vi "Stop Data Grid.vi"(8 "error in (no error)":errorcluster, 11 "DataGridView in":refnum<class "DataGridView.lvclass">) -> (0 "error out":errorcluster, 3 "DataGridView out":refnum<class "DataGridView.lvclass">)   [LabVIEW 2016, in "DataGrid.lvlib" / "DataGridView.lvclass"]
doc: "This VI must be called to properly stop the grid, as it unregisters the .net callback events, that otherwise, stay running and lock the classes."
uses:
  <userlib>/LabVIEWdotNetDataGrid/source/DataGridView/DataGridView.lvclass
  <userlib>/LabVIEWdotNetDataGrid/source/DataGridView/DataGridView.lvclass/DataGridView.ctl
  System.Windows.Forms
  <userlib>/LabVIEWdotNetDataGrid/source/DataTable/DataTable.lvclass/DataTable.ctl
  System.Data
  <userlib>/LabVIEWdotNetDataGrid/source/DataTable/Read DataTable.vi
  <userlib>/LabVIEWdotNetDataGrid/source/DataTable/DataTable.lvclass
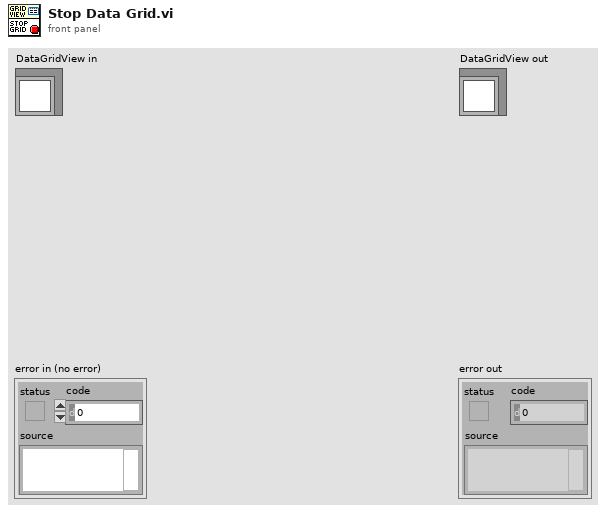
[diagram p1: front panel]
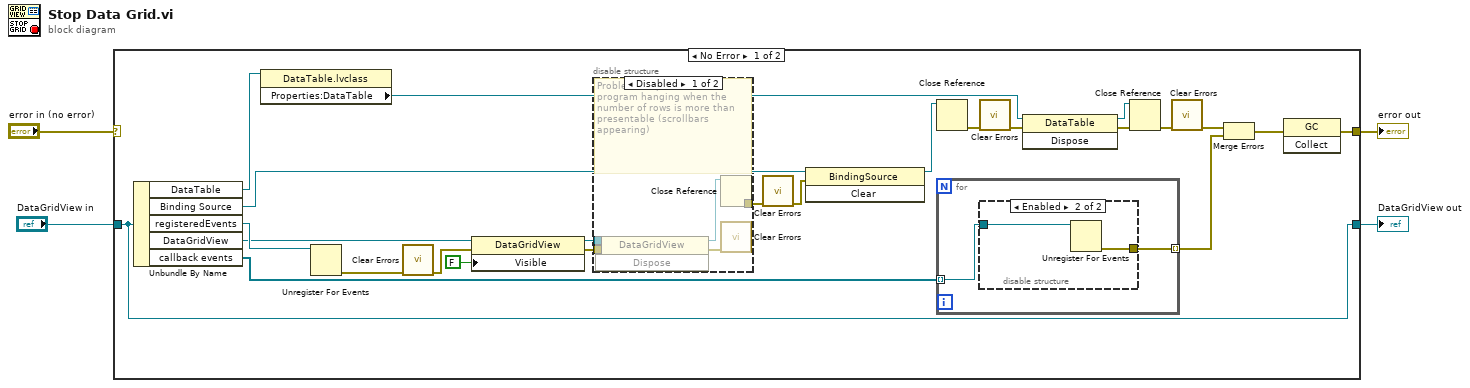
[diagram p0: block diagram]
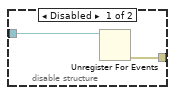
[diagram p3: hidden frame]
diagram:
  n1 = case shown="No Error" "error in (no error)" {
    selector: "error in (no error)" -> [_ w42]
    tunnel: [w24 w42] -> w3
    tunnel: [w28 w41] -> w1
    tunnel: "DataGridView in" -> [w28 w41]
    frame No Error {
      n2 = Unbundle By Name(w28) -> ("DataTable"=w23:refnum<class "DataTable.lvclass">, "Binding Source"=w20:refnum<k24>, "registeredEvents"=w22:refnum<event-registration>, "DataGridView"=w21:refnum<k24>, "callback events"=w27:refnum<k27>[])
      n3 = property class="DataTable.lvclass"(reference=w23) -> ("Properties:DataTable"=w19:refnum<k24>)  [unwired: 1 in, 2 out]
      n4 = Unregister For Events(event registration refnum=w22) -> (error out=w16:errorcluster)  [unwired: 1 in]
      n5 = call <vilib>:"Clear Errors.vi"("error in (no error)"=w16) -> ("error out"=w6:errorcluster)  [unwired: 5 in, 1 out]
      n6 = property class="DataGridView"(reference=w21, error in=w6, "Visible"=FALSE) -> (reference out=w14:refnum<k24>, error out=w13:errorcluster)
      n7 = disable-structure shown="Disabled" {
        disable-tunnel: w14 -> [w32 _]
        disable-tunnel: w13 -> [w31 w34]
        disable-tunnel: [w30 w34] -> w12
        frame Disabled {
          # "Problem: dispose causes program hanging when the number of rows is more than presentable (scrollbars appearing)"
          n8 = invoke class="DataGridView" method="Dispose"(reference=w32, error in=w31) -> (reference out=w33:refnum<k24>, error out=w29:errorcluster)  [unwired: 1 in, 1 out]
          n9 = Close Reference(reference=w33) -> (error out=w30:errorcluster)  [unwired: 1 in]
          n10 = call <vilib>:"Clear Errors.vi"("error in (no error)"=w29) -> ()  [unwired: 5 in, 2 out]
        }
        frame Enabled {
        }
      }
      n11 = call <vilib>:"Clear Errors.vi"("error in (no error)"=w12) -> ("error out"=w18:errorcluster)  [unwired: 5 in, 1 out]
      n12 = invoke class="BindingSource" method="Clear"(reference=w20, error in=w18) -> (reference out=w11:refnum<k24>)  [unwired: 1 in, 2 out]
      n13 = Close Reference(reference=w11) -> (error out=w10:errorcluster)  [unwired: 1 in]
      n14 = for {
        tunnel: w27 -> [w36] mode=indexing
        tunnel: [w35] -> w26 mode=indexing
        n15 = disable-structure shown="Enabled" {
          disable-tunnel: w36 -> [w38 w40]
          disable-tunnel: [w37 w39] -> w35
          frame Disabled {
            n16 = Unregister For Events(event registration refnum=w38) -> (error out=w37:errorcluster)  [unwired: 1 in]
          }
          frame Enabled {
            n17 = Unregister For Events(event registration refnum=w40) -> (error out=w39:errorcluster)  [unwired: 1 in]
          }
        }
      }
      n18 = call <vilib>:"Clear Errors.vi"("error in (no error)"=w10) -> ("error out"=w17:errorcluster)  [unwired: 5 in, 1 out]
      n19 = invoke class="DataTable" method="Dispose"(reference=w19, error in=w17) -> (reference out=w7:refnum<k24>, error out=w9:errorcluster)  [unwired: 1 in, 1 out]
      n20 = Close Reference(reference=w7, error in (no error)=w9) -> (error out=w8:errorcluster)
      n21 = call <vilib>:"Clear Errors.vi"("error in (no error)"=w8) -> ("error out"=w5:errorcluster)  [unwired: 5 in, 1 out]
      n22 = Merge Errors(w5, w26) -> (w25:errorcluster)
      n23 = invoke class="GC" method="Collect"(error in=w25) -> (error out=w24:errorcluster)  [unwired: 2 in, 2 out]
    }
    frame Error {
    }
  }
  "error out" <- w3
  "DataGridView out" <- w1
